vi "FRCts20_Backend_LinearSearchTeamNumber.vi"(8 "error in (no error)":errorcluster, 9 "Team Number":u16, 11 "Competitions":T1) -> (0 "error out":errorcluster, 1 "Index":i32, 2 "Found?":bool, 3 "Competitions Oot":T1)   [LabVIEW 2014, in "FRCts20_Backend_Engine_Deprecated.lvlib"]
uses:
  FRCts20_Backend_Engine_Deprecated.lvlib
  FRCts20_Backend_TeamDataDfn.ctl
  FRCts20_Backend_Controls.lvlib
  FRCts20_Backend_TeamDfn.ctl
  FRCts20_Backend_IssueDfn.ctl
  FRCts20_Backend_Team_Info.ctl
  FRCts20_Backend_Note.ctl
  FRCts20_Backend_Note_list.ctl
  FRCts20_Backend_request_info.ctl
  FRCts20_Backend_IssueTeamList.ctl
  FRCts20_Backend_Competition_Info.ctl
  FRCts20_Backend_Division_Info.ctl
  FRCts20_Backend_Division.ctl
  FRCts20_Backend_Division_List.ctl
  FRCts20_Backend_Competition.ctl
  FRCts20_Backend_Competition_List.ctl
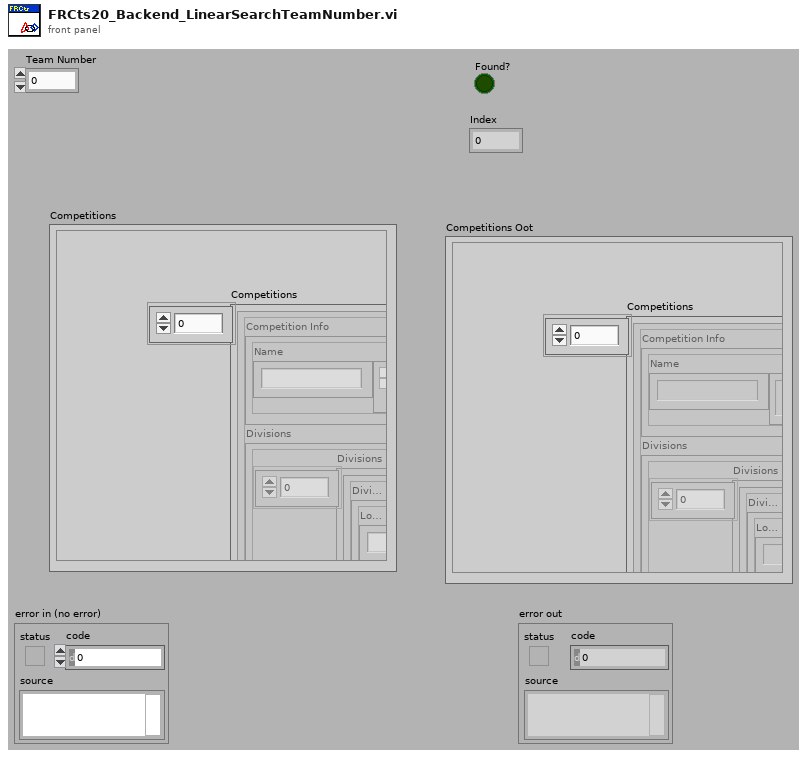
[diagram p1: front panel]
types:
  T1 = typedef "FRCts20_Backend_Controls.lvlib/FRCts20_Backend_Competition_List.ctl" = cluster{"Competitions":T2[]}
  T2 = typedef "FRCts20_Backend_Controls.lvlib/FRCts20_Backend_Competition.ctl" = cluster{"Competition Info":T3, "Divisions":T4}
  T3 = typedef "FRCts20_Backend_Controls.lvlib/FRCts20_Backend_Competition_Info.ctl" = cluster{"Name":string, "Start Date":timestamp, "Duration":u8}
  T4 = typedef "FRCts20_Backend_Controls.lvlib/FRCts20_Backend_Division_List.ctl" = cluster{"Divisions":T5[]}
  T5 = typedef "FRCts20_Backend_Controls.lvlib/FRCts20_Backend_Division.ctl" = cluster{"Division Info":T6, "TeamData":T7}
  T6 = typedef "FRCts20_Backend_Controls.lvlib/FRCts20_Backend_Division_Info.ctl" = cluster{"Location":string}
  T7 = typedef "FRCts20_Backend_Controls.lvlib/FRCts20_Backend_TeamDataDfn.ctl" = cluster{"Team":T8[]}
  T8 = typedef "FRCts20_Backend_Controls.lvlib/FRCts20_Backend_TeamDfn.ctl" = cluster{"Team Info":T9, "IssueList":T10}
  T9 = typedef "FRCts20_Backend_Controls.lvlib/FRCts20_Backend_Team_Info.ctl" = cluster{"TeamNumber":u16, "SWType":string}
  T10 = typedef "FRCts20_Backend_Controls.lvlib/FRCts20_Backend_IssueTeamList.ctl" = cluster{"Issues":T11[]}
  T11 = typedef "FRCts20_Backend_Controls.lvlib/FRCts20_Backend_IssueDfn.ctl" = cluster{"Notes":T12, "Info":T14}
  T12 = typedef "FRCts20_Backend_Controls.lvlib/FRCts20_Backend_Note_list.ctl" = cluster{"Notes":T13[]}
  T13 = typedef "FRCts20_Backend_Controls.lvlib/FRCts20_Backend_Note.ctl" = cluster{"Time Entered":timestamp, "Author":string, "Text":string}
  T14 = typedef "FRCts20_Backend_Controls.lvlib/FRCts20_Backend_request_info.ctl" = cluster{"Status":enum16{"Open", "In Work", "Closed"}, "Open Date":timestamp, "Description":string, "Last Update":timestamp, "Closed Date":timestamp, "Solution Index":i32}
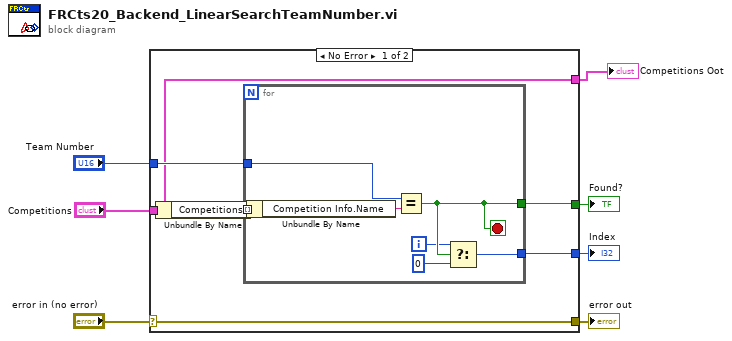
[diagram p0: block diagram]
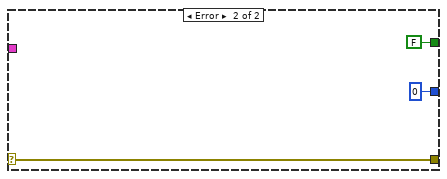
[diagram p2: hidden frame]
diagram:
  n1 = case shown="No Error" "error in (no error)" {
    selector: "error in (no error)" -> [w9 w23]
    tunnel: [w9 w23] -> w6
    tunnel: "Competitions" -> [w8 _]
    tunnel: "Team Number" -> [w12 _]
    tunnel: [w11 FALSE] -> w4
    tunnel: [w10 0 ("f")] -> w3
    tunnel: [w8 _] -> w1
    frame No Error {
      n2 = Unbundle By Name(w8) -> ("Competitions"=w13:T2[])
      n3 = for {
        tunnel: w13 -> [w20] mode=indexing
        tunnel: w12 -> [w18]
        tunnel: [w17] -> w11
        tunnel: [w14] -> w10
        i -> [w16]
        stop <- w17 stop-if-true
        n4 = Unbundle By Name(w20) -> ("Competition Info.Name"=w19:string)
        n5 = Equal?(x=w18, y=w19) -> (x = y?=w17:bool)
        n6 = Select(t=w16, s=w17, f=0) -> (s? t:f=w14:i32)
      }
    }
    frame Error {
    }
  }
  "error out" <- w6
  "Found?" <- w4
  "Index" <- w3
  "Competitions Oot" <- w1
